vi "Close.vi"(8 "error in (no error)":errorcluster, 11 "Data in":refnum<class "Const_WFM.lvclass">) -> (0 "error out":errorcluster, 3 "Data out":refnum<class "Const_WFM.lvclass">)   [LabVIEW 2021, in "Const_WFM.lvclass"]
uses:
  Const_WFM.lvclass
  Const_WFM.lvclass/Const_WFM.ctl
  Abs_Types/Waveform/Abs_Waveform.lvclass
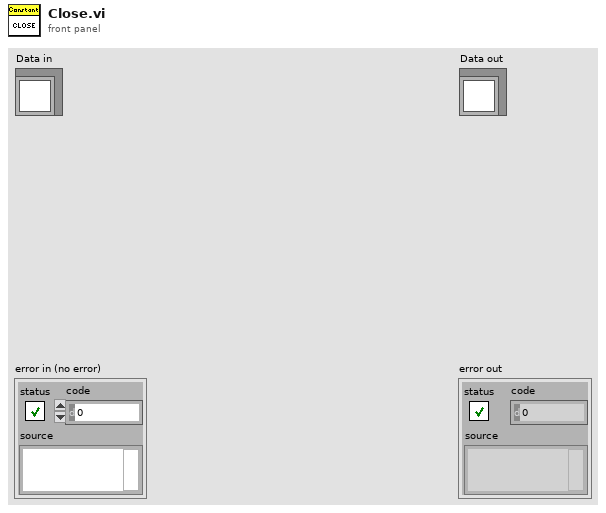
[diagram p1: front panel]
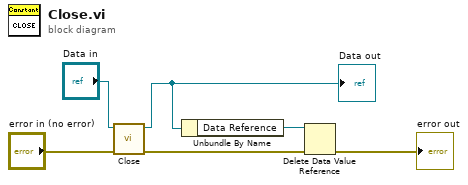
[diagram p0: block diagram]
diagram:
  n1 = call-parent "Close.vi"("error in (no error)"="error in (no error)", "Data in"="Data in") -> ("error out"=w3:errorcluster, "Data out"=w4:refnum<class "Const_WFM.lvclass">)  [unwired: 8 in]
  "Data out" <- w4
  n2 = Unbundle By Name(w4) -> ("Data Reference"=w2:refnum<data-value>)
  n3 = Delete Data Value Reference(data value reference=w2, error in=w3) -> (error out=→"error out":errorcluster)  [unwired: 1 out]
